vi "Poisson Noise (obs 90).vi"(2 "seed":i32=-1, 3 "mean":dbl=1.0 format="%0.2f", 4 "samples":i32=128) -> (0 "error":i32, 1 "poisson noise":dbl[](array[numeric]))   [LabVIEW 2010, in "NI_AALBase.lvlib"]
doc: "The Poisson Noise VI was rewritten in LabVIEW 2009. Replace this VI with a Poisson Noise VI from the <B>Functions</B> palette to use the new functionality.\n\nGenerates a pseudorandom sequence of values that are the number of discrete events occurring in a given interval, specified by <B>mean</B>, of a unit rate Poisson process."
uses:
  NI_AALBase.lvlib
  lvanlys.dll
panel:
  # "Poisson Noise"
  # "This VI is obsolete !!!\nYou should replace this VI in your diagram with the Poisson Noise VI."
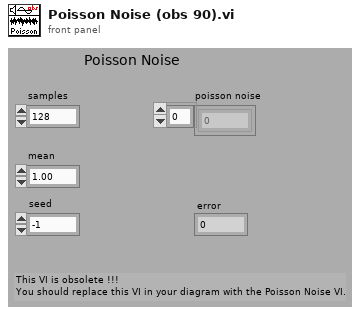
[diagram p1: front panel]
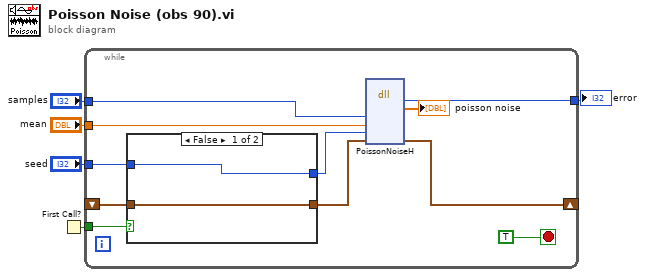
[diagram p0: block diagram]
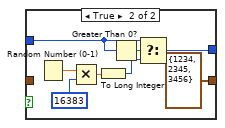
[diagram p2: hidden frame]
diagram:
  n1 = First Call?() -> (First Call?: T/F=w1:bool)
  n2 = while {
    tunnel: [w12] -> w5
    tunnel: "seed" -> [w10]
    tunnel: "mean" -> [w16]
    tunnel: "samples" -> [w15]
    shift-right: [w11] -> _
    shift-left: _ -> [w8]
    tunnel: w1 -> [w6]
    stop <- TRUE stop-if-true
    n3 = case shown="False" w6 {
      tunnel: w8 -> [w18 _]
      tunnel: [w18 cluster{"xSeed":i32, "ySeed":i32, "zSeed":i32} {"xSeed"=1234, "ySeed"=2345, "zSeed"=3456} ("RNGState")] -> w7
      tunnel: [w17 w24] -> w9
      tunnel: w10 -> [w17 w25]
      frame False {
      }
      frame True {
        n4 = Random Number (0-1)() -> (number: 0 to 1=w22:dbl)
        n5 = Multiply(x=w22, y=16383 ("x")) -> (x*y=w23:dbl)
        n6 = To Long Integer(number=w23) -> (32bit integer=w21:i32)
        n7 = Greater Than 0?(x=w25) -> (x > 0?=w26:bool)
        n8 = Select(t=w25, s=w26, f=w21) -> (s? t:f=w24:i32)
      }
    }
    n9 = dll-call lib="C:/Program Files/National Instruments/LabVIEW 2010/resource/lvanlys.*" fn="PoissonNoiseH"("size"=w15, "mean"=w16, "theSeed"=w9, "rngState"=w7) -> ("return type"=w12:i32, "poisson noise"=→"poisson noise":dbl[], "rngState"=w11:cluster{"xSeed":i32, "ySeed":i32, "zSeed":i32})  [unwired: 6 in, 3 out]
  }
  "error" <- w5
